vi "bytearray2frame.vi"(1 "CAN template":T1 {"payload" format="%x"; "timestamp" format="%<%.7X\n%x>T"; "type" items=["CAN Data"=0, "CAN Remote"=1, "CAN Bus Error"=2, "CAN 2.0 Data"=8, "CAN FD Data"=16, "CAN FD+BRS Data"=24, "J1939 Data"=192, "Delay"=224, "Log Trigger"=225, "Start Trigger"=226]; "identifier" format="%x"}, 2 "2D Array":u8[][](array[numeric])) -> (0 "CAN frame array":T1[](array[typedef]) {"payload" format="%x"; "timestamp" format="%<%.7X\n%x>T"; "type" items=["CAN Data"=0, "CAN Remote"=1, "CAN Bus Error"=2, "CAN 2.0 Data"=8, "CAN FD Data"=16, "CAN FD+BRS Data"=24, "J1939 Data"=192, "Delay"=224, "Log Trigger"=225, "Start Trigger"=226]; "identifier" format="%x"})   [LabVIEW 2017]
uses:
  <vilib>/xnet/xnet.llb/XNET Frame CAN.ctl
  <vilib>/xnet/xnet.llb/XNET Frame Type CAN.ctl
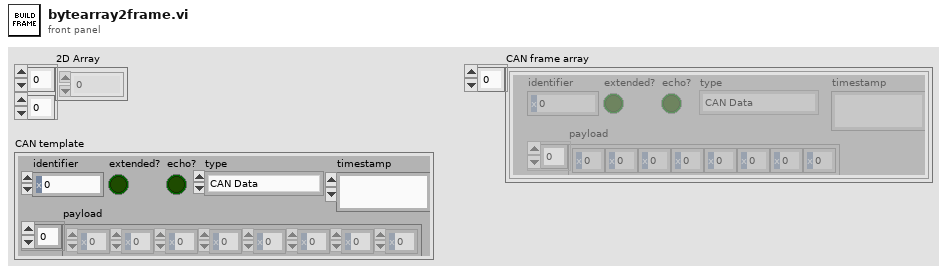
[diagram p1: front panel]
types:
  T1 = typedef "XNET Frame CAN.ctl" = cluster{"timestamp":timestamp, "payload":u8[], "identifier":u32, "type":T2, "extended?":bool, "echo?":bool}
  T2 = typedef "XNET Frame Type CAN.ctl" = u8
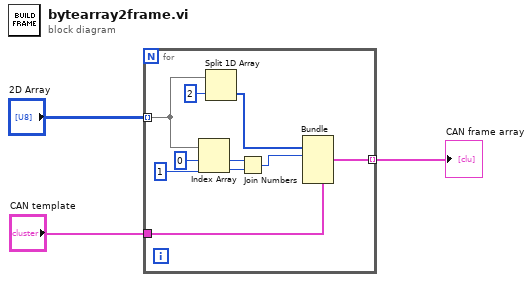
[diagram p0: block diagram]
diagram:
  n1 = for {
    tunnel: "2D Array" -> [w9] mode=indexing
    tunnel: [w5] -> w2 mode=indexing
    tunnel: "CAN template" -> [w4]
    n2 = Index Array(array=w9, index #1=0 ("index"), index #2=1 ("index")) -> (element #1=w11:u8, element #2=w10:u8)
    n3 = Split 1D Array(array=w9, index=2) -> (second subarray=w7:u8[])  [unwired: 1 out]
    n4 = Join Numbers(hi=w11, lo=w10) -> ((hi.lo)=w6:u16)
    n5 = Bundle(cluster=w4, "payload"=w7, "identifier"=w6) -> (w5:T1)  [unwired: 4 in]
  }
  "CAN frame array" <- w2
